vi "Search 1D Array (SGL)__ogtk.vi"(0 "Array":sgl[](array[numeric]) format="%.2f", 2 "Element Data":sgl format="%.2f", 3 "Start Index (0)":i32) -> (7 "Indices of Elements":i32[](array[numeric]))   [LabVIEW 2020]
doc: "Searches for all element data matches in array"
panel:
  # "[OpenG VI Tags] ***Do Not Remove***\n\nSVN Revision = 990\nSVN Revision Date = 2009-07-18 07:14:13 -0700 (Sat, 18 Jul 2009)\nPackage = oglib_array-3.0.0-1\nDepends ="
  # "Search 1D Array.vi\n\nSearches for all element data matches in array\n\nPlease visit http://www.OpenG.org to learn about the\nOpen Source LabVIEW software movement.\n\nNOTICE -- YOU MUST LEAVE THIS NOTICE IN PLACE.  PER THE TERMS OF THE LICENSE BELOW, YOU MAY SUBLICENSE THIS SOFTWARE \nIN ANY WAY THAT DOES NOT CONFLICT WITH THIS LICENSE.\n\n### BSD License (http://www.opensource.org/licenses/bsd-license.php) Begin ###\n \nCopyright (c) 2005, MKS Instruments, Inc., author: Doug Femec<doug_femec@mksinst.com>, IM dafemec\n\nAll rights reserved.\n\nRedistribution and use in source and binary forms, with or without modification, are permitted provided that the following conditions are met:\n\n    * Redistributions of source code must retain the above copyright notice, this list of conditions and the following disclaimer.\n    * Redistributions in binary form must reproduce the above copyright notice, this list of conditions and the following disclaimer in the \n       documentation and/or other materials provided with the distribution.\n    * Neither the name of SciWare, James Kring, Inc., nor the names of its contributors may be used to endorse or promote products derived \n       from this software without specific prior written permission.\n\nTHIS SOFTWARE IS PROVIDED BY THE COPYRIGHT HOLDERS AND CONTRIBUTORS \"AS IS\" AND ANY EXPRESS OR IMPLIED WARRANTIES, \nINCLUDING, BUT NOT LIMITED TO, THE IMPLIED WARRANTIES OF MERCHANTABILITY AND FITNESS FOR A PARTICULAR PURPOSE ARE \nDISCLAIMED. IN NO EVENT SHALL THE COPYRIGHT OWNER OR CONTRIBUTORS BE LIABLE FOR ANY DIRECT, INDIRECT, INCIDENTAL,\n SPECIAL, EXEMPLARY, OR CONSEQUENTIAL DAMAGES (INCLUDING, BUT NOT LIMITED TO, PROCUREMENT OF SUBSTITUTE GOODS OR \nSERVICES; LOSS OF USE, DATA, OR PROFITS; OR BUSINESS INTERRUPTION) HOWEVER CAUSED AND ON ANY THEORY OF LIABILITY, \nWHETHER IN CONTRACT, STRICT LIABILITY, OR TORT (INCLUDING NEGLIGENCE OR OTHERWISE) ARISING IN ANY WAY OUT OF THE USE \nOF THIS SOFTWARE, EVEN IF ADVISED OF THE POSSIBILITY OF SUCH DAMAGE.\n\n### BSD License End ###"
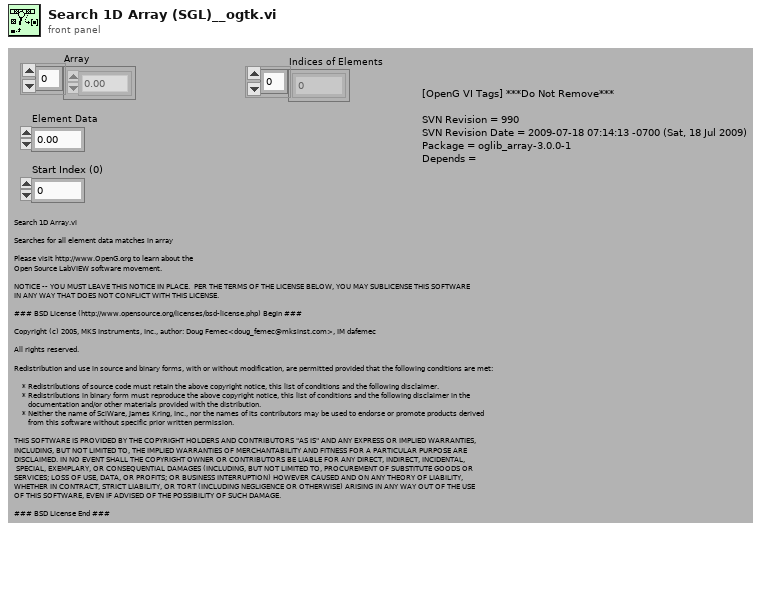
[diagram p1: front panel]
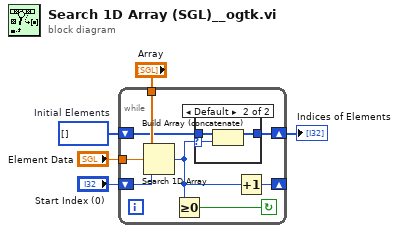
[diagram p0: block diagram]
diagram:
  w1 = i32[] []  # Initial Elements
  n1 = while {
    shift-right: [w6] -> _
    shift-left: "Start Index (0)" -> [w13]
    shift-right: [w10] -> w5
    shift-left: w1 -> [w11]
    tunnel: "Array" -> [w12]
    tunnel: "Element Data" -> [w9]
    stop <- w7 continue-if-true
    n2 = Search 1D Array(1D array=w12, element=w9, start index (0)=w13) -> (index of element=w8:i32)
    n3 = Greater Or Equal To 0?(x=w8) -> (x >= 0?=w7:bool)
    n4 = case shown="Default" w8 {
      selector: w8 -> [_ w17]
      tunnel: w11 -> [w14 w16]
      tunnel: [w14 w15] -> w10
      frame -1 {
      }
      frame Default {
        n5 = Build Array (concatenate)(w16, w17) -> (w15:i32[])
      }
    }
    n6 = Increment(x=w8) -> (x+1=w6:i32)
  }
  "Indices of Elements" <- w5
